vi "PQclose.vi"(8 "error in (no error)":errorcluster, 11 "conn":u32) -> (0 "error out":errorcluster)   [LabVIEW 2019, in "libpqutility.lvlib"]
doc: "Disconnect from PostgreSQL database.\nSee PostgreSQL c-lib doku for further information."
uses:
  libpqutility.lvlib
  libpqlv/libpqlv.lvlib
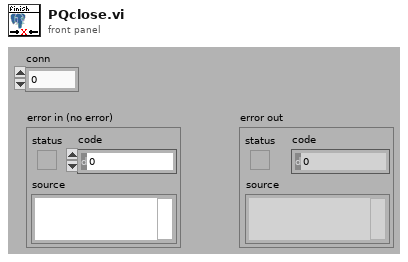
[diagram p1: front panel]
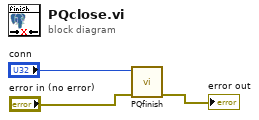
[diagram p0: block diagram]
diagram:
  n1 = call "PQfinish.vi"("error in (no error)"="error in (no error)", "conn"="conn") -> ("error out"=→"error out":errorcluster)  [unwired: 9 in]
